vi "Climber State Control.vi"(11 "Desired Position":dbl) -> ()   [LabVIEW 2012]
uses:
  FRC_2013_Labview_Project/Ultimate Ascent/Robot Global Data.vi
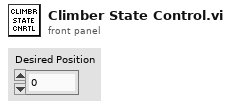
[diagram p1: front panel]
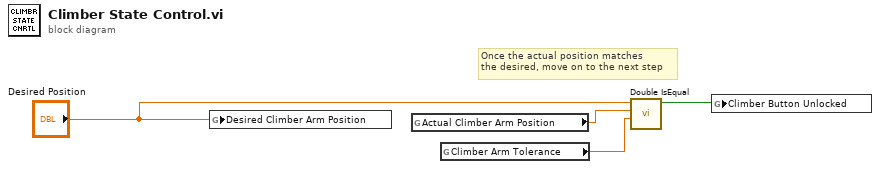
[diagram p0: block diagram]
diagram:
  # "Once the actual position matches\nthe desired, move on to the next step"
  n1 = global write "Robot Global Data.vi" "Desired Climber Arm Position"("Desired Position") -> ()
  n2 = global read "Robot Global Data.vi" "Actual Climber Arm Position"() -> (w4:dbl)
  n3 = global read "Robot Global Data.vi" "Climber Arm Tolerance"() -> (w3:dbl)
  n4 = call "Double IsEqual.vi"("Epsilon"=w3, "Double2"=w4, "Double1"="Desired Position") -> ("IsEqual"=w1:bool)  [unwired: 8 in]
  n5 = global write "Robot Global Data.vi" "Climber Button Unlocked"(w1) -> ()
